vi "Edgertronic-:dir_listing copy.vi"(5 "Setup":T2={"URL"="130.64.16.195", "remote port"=80, "mode (standard)"=enum."Standard"}) -> (0 "error out":errorcluster, 1 "Directory Listing:":T1, 2 "data out":string="HTTP/1.0 200 OK\r\nContent-Type: text/html; charset=utf-8\r\nContent-Length: 313\r\nConnection: close\r\nDate: Tue, 16 Jun 2015 13:54:12 GMT\r\nServer: lighttpd/1.4.11 (edgertonic slow motion camera)\r\n\r\n{\"build_date\": \"20150112\", \"sw_build_date\": \"20140911165611\", \"fpga_initialized\": 1, \"hardware_revision\": 6, \"model_number\": 1, \"home_dir\": \"/home/root/ss-web\", \"ir_filter\": 1, \"mac_addr\": \"00:1B:C5:09:61:4D\", \"serial_console_enabled\": false, \"serial_number\": 333, \"fpga_version\": 70, \"hardware_configuration\": 1}")   [LabVIEW 2012]
doc: "This VI returns the list of files in the active storage video directory."
panel:
  in  "GET Cmd":string="/dir_listing"
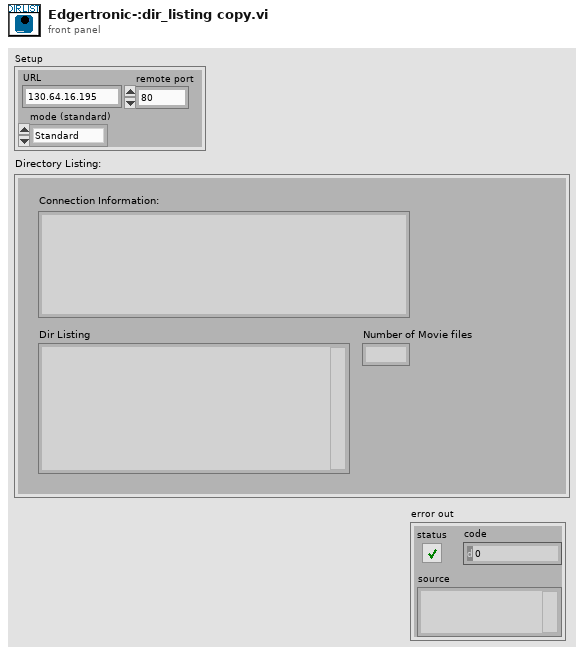
[diagram p1: front panel]
types:
  T1 = cluster{"Connection Information:":string, "Dir Listing":string, "Number of Movie files":string}
  T2 = cluster{"URL":string, "remote port":u16, "mode (standard)":enum16{"Standard", "Buffered", "CRLF", "Immediate"}}
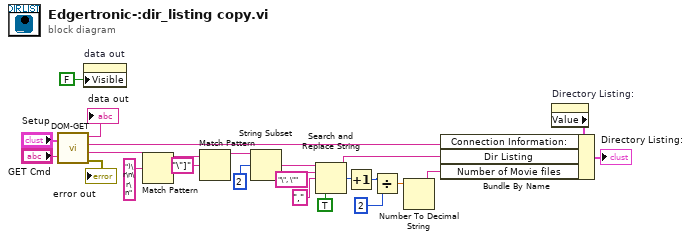
[diagram p0: block diagram]
diagram:
  n1 = call <userlib>:"DOM-GET.vi"("Setup"="Setup", "GET Command"="GET Cmd") -> ("Data Out from Camera"=→"data out":string, "Connection Information"=w3:string, "Value String"=w2:string, "error out"=→"error out":errorcluster)
  n2 = property on="data out" class="Str"("Visible"=FALSE) -> ()  [unwired: 2 in, 2 out]
  n3 = Match Pattern(string=w2, regular expression=")\r\n\r\n") -> (before substring=w4:string)  [unwired: 1 in, 3 out]
  n4 = Match Pattern(string=w4, regular expression="\"]") -> (before substring=w18:string)  [unwired: 1 in, 3 out]
  n5 = String Subset(string=w18, offset (0)=2) -> (substring=w16:string)  [unwired: 1 in]
  n6 = Search and Replace String(replace all?=TRUE ("replace all? (F)"), input string=w16, search string="\", \"" ("regular expression (\"\")"), replace string="," ("replace string (\"\")")) -> (result string=w5:string, number of replacements=w12:i32)  [unwired: 4 in, 2 out]
  n7 = Increment(x=w12) -> (x+1=w10:i32)
  n8 = Divide(x=w10, y=2) -> (x/y=w7:dbl)
  n9 = Number To Decimal String(number=w7) -> (decimal integer string=w6:string)  [unwired: 1 in]
  n10 = property on="Directory Listing:" class="Clust (strict)"() -> ("Value"=w1:T1)  [unwired: 2 in, 2 out]
  n11 = Bundle By Name(cluster=w1, "Connection Information:"=w3, "Dir Listing"=w5, "Number of Movie files"=w6) -> (→"Directory Listing:":T1)
